vi "Le_string_fram.vi"() -> ()   [LabVIEW 2019]
panel:
  in  "STRING 2":string
  out "STRING":string
  in  "MWU2987":i16
  in  "MWU2976":i16
  in  "MWU2975":i16
  in  "MWU2986":i16
  in  "MWU2977":i16
  in  "MWU2978":i16
  in  "MWU2979":i16
  in  "MWU2981":i16
  in  "MWU2982":i16
  in  "MWU2983":i16
  in  "MWU2980":i16
  in  "MWU2984":i16
  in  "MWU2985":i16
  in  "STOP":bool
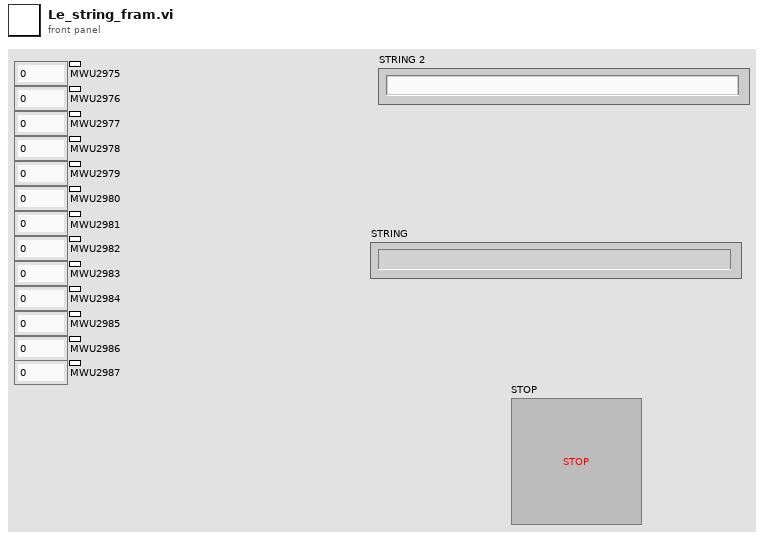
[diagram p1: front panel]
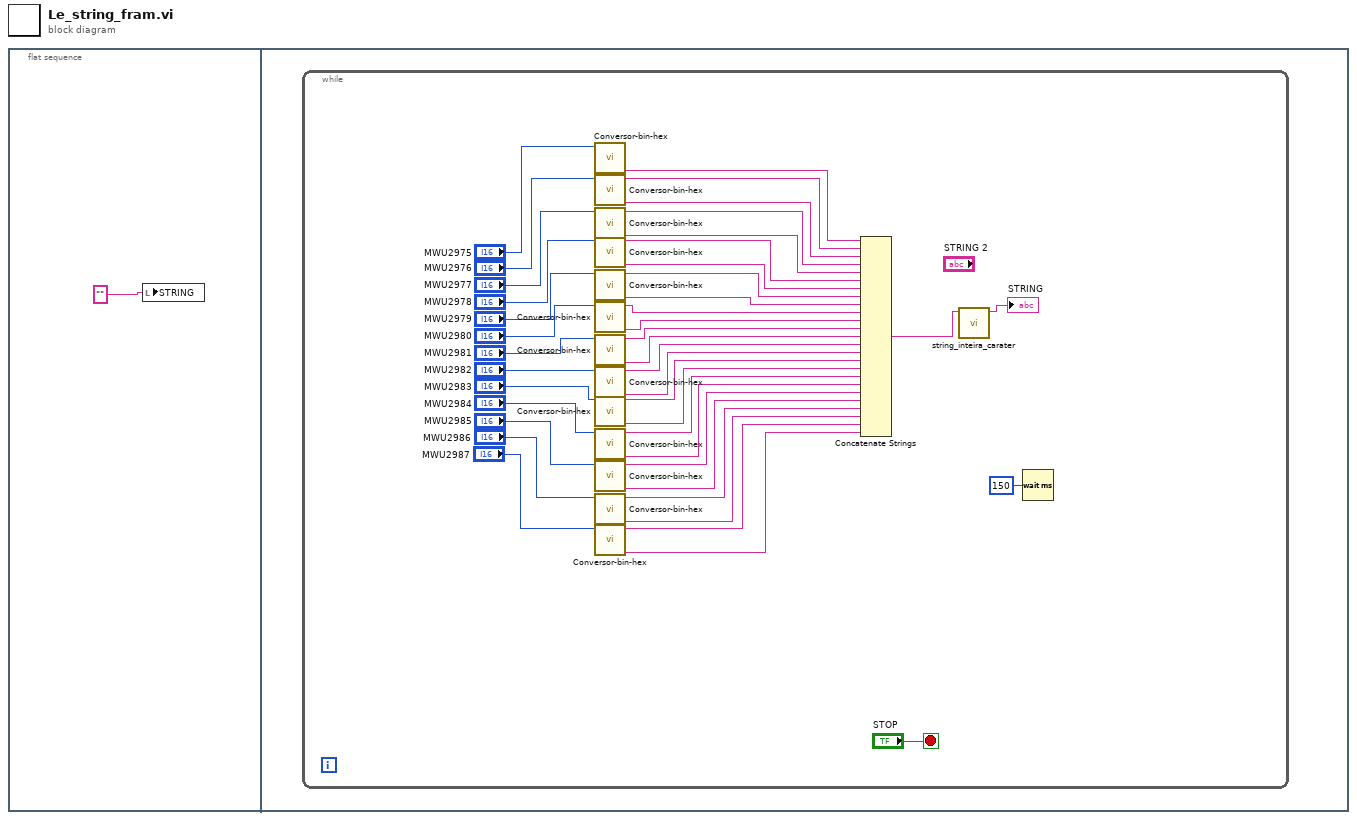
[diagram p0: block diagram]
diagram:
  n1 = flat-sequence {
    frame #0 {
      n2 = local write "STRING"("" ("STRING")) -> ()
    }
    frame #1 {
      n3 = while {
        stop <- "STOP" stop-if-true
        n4 = call "Conversor-bin-hex.vi"("Numeric"="MWU2975") -> ("hex integer string"=w30:string)  [unwired: 9 in, 1 out]
        n5 = call "Conversor-bin-hex.vi"("Numeric"="MWU2976") -> ("hex integer string"=w28:string, "hex integer string 2"=w29:string)  [unwired: 9 in]
        n6 = call "Conversor-bin-hex.vi"("Numeric"="MWU2977") -> ("hex integer string"=w26:string, "hex integer string 2"=w27:string)  [unwired: 9 in]
        n7 = call "Conversor-bin-hex.vi"("Numeric"="MWU2978") -> ("hex integer string"=w24:string, "hex integer string 2"=w25:string)  [unwired: 9 in]
        n8 = call "Conversor-bin-hex.vi"("Numeric"="MWU2979") -> ("hex integer string"=w22:string, "hex integer string 2"=w23:string)  [unwired: 9 in]
        n9 = call "Conversor-bin-hex.vi"("Numeric"="MWU2980") -> ("hex integer string"=w20:string, "hex integer string 2"=w21:string)  [unwired: 9 in]
        n10 = call "Conversor-bin-hex.vi"("Numeric"="MWU2981") -> ("hex integer string"=w18:string, "hex integer string 2"=w19:string)  [unwired: 9 in]
        n11 = call "Conversor-bin-hex.vi"("Numeric"="MWU2982") -> ("hex integer string"=w16:string, "hex integer string 2"=w17:string)  [unwired: 9 in]
        n12 = call "Conversor-bin-hex.vi"("Numeric"="MWU2983") -> ("hex integer string"=w14:string, "hex integer string 2"=w15:string)  [unwired: 9 in]
        n13 = call "Conversor-bin-hex.vi"("Numeric"="MWU2984") -> ("hex integer string"=w12:string, "hex integer string 2"=w13:string)  [unwired: 9 in]
        n14 = call "Conversor-bin-hex.vi"("Numeric"="MWU2985") -> ("hex integer string"=w10:string, "hex integer string 2"=w11:string)  [unwired: 9 in]
        n15 = call "Conversor-bin-hex.vi"("Numeric"="MWU2986") -> ("hex integer string"=w8:string, "hex integer string 2"=w9:string)  [unwired: 9 in]
        n16 = call "Conversor-bin-hex.vi"("Numeric"="MWU2987") -> ("hex integer string"=w5:string, "hex integer string 2"=w6:string)  [unwired: 9 in]
        n17 = Concatenate Strings(w30, w29, w28, w27, w26, w25, w24, w23, w22, w21, w20, w19, w18, w17, w16, w15, w14, w13, w12, w11, w10, w9, w8, w6, w5) -> (w4:string)
        n18 = call "string_inteira_carater.vi"("String in"=w4) -> ("String out"=→"STRING":string)  [unwired: 10 in]
        n19 = Wait (ms)(milliseconds to wait=u32 150) -> ()  [unwired: 1 out]
      }
    }
  }
